vi "Pulse once on press.vi"(0 "in":bool, 1 "duration of pulse":dbl) -> (6 "pulse":bool)   [LabVIEW 2017]
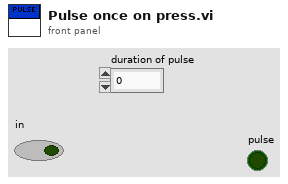
[diagram p1: front panel]
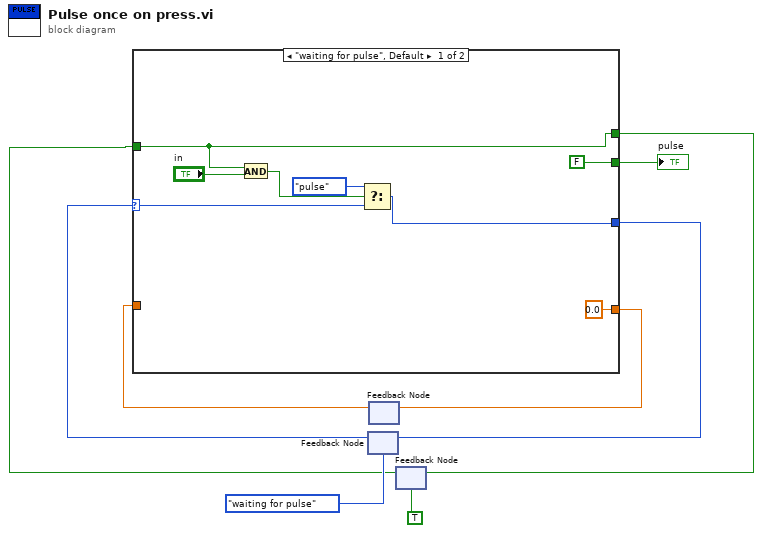
[diagram p0: block diagram]
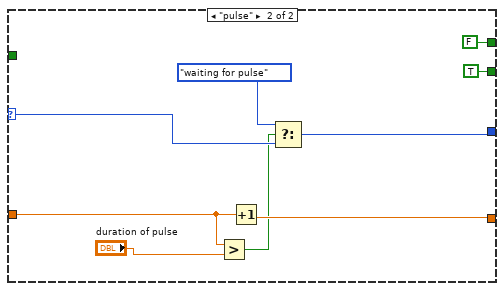
[diagram p2: hidden frame]
diagram:
  n1 = feedback #1(enum16{"waiting for pulse", "pulse"}."waiting for pulse") -> (w8:enum16{"waiting for pulse", "pulse"})
  n2 = feedback #2() -> (w4:dbl)  [unwired: 1 in]
  n3 = feedback #3(TRUE) -> (w2:bool)
  n4 = case shown="\"waiting for pulse\", Default" w8 {
    selector: w8 -> [w17 w24]
    tunnel: [w16 w25] -> w9
    tunnel: [FALSE TRUE] -> w6
    tunnel: w4 -> [_ w21]
    tunnel: [0.0 w22] -> w5
    tunnel: [w11 FALSE] -> w3
    tunnel: w2 -> [w11 _]
    frame "waiting for pulse", Default {
      n5 = And(x=w11, y="in") -> (x .and. y?=w13:bool)
      n6 = Select(t=enum16{"waiting for pulse", "pulse"}."pulse", s=w13, f=w17) -> (s? t:f=w16:enum16{"waiting for pulse", "pulse"})
    }
    frame "pulse" {
      n7 = Greater?(x=w21, y="duration of pulse") -> (0:w19:bool)
      n8 = Increment(x=w21) -> (x+1=w22:dbl)
      n9 = Select(t=enum16{"waiting for pulse", "pulse"}."waiting for pulse", s=w19, f=w24) -> (s? t:f=w25:enum16{"waiting for pulse", "pulse"})
    }
  }
  "pulse" <- w6
  n10 = feedback-in #1(w9) -> ()
  n11 = feedback-in #2(w5) -> ()
  n12 = feedback-in #3(w3) -> ()
